vi "仪器初始化.vi"(8 "错误输入（无错误）":errorcluster, 11 "仪器地址":T1) -> (0 "error out":errorcluster, 3 "仪器实例 out":T2)   [LabVIEW 2021]
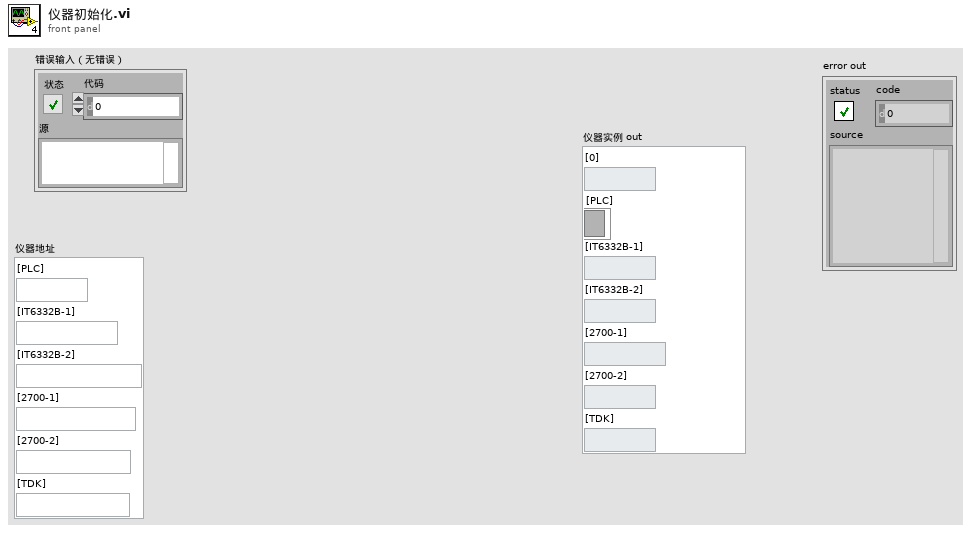
[diagram p1: front panel]
types:
  T1 = typedef "仪器地址输入.ctl" = cluster{"[PLC]":string, "[IT6332B-1]":string, "[IT6332B-2]":string, "[2700-1]":string, "[2700-2]":string, "[TDK]":string}
  T2 = typedef "仪器实例.ctl" = cluster{"[0]":string, "[PLC]":refnum<k24>, "[IT6332B-1]":string, "[IT6332B-2]":string, "[2700-1]":string, "[2700-2]":string, "[TDK]":string}
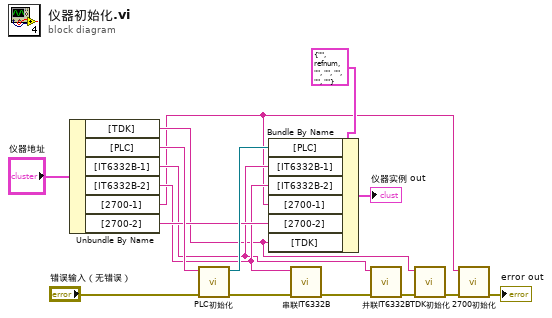
[diagram p0: block diagram]
diagram:
  n1 = Unbundle By Name("仪器地址") -> ("[TDK]"=w5:string, "[PLC]"=w13:string, "[IT6332B-1]"=w7:string, "[IT6332B-2]"=w8:string, "[2700-1]"=w1:string, "[2700-2]"=w10:string)
  n2 = call "PLC初始化.vi"("错误输入（无错误）"="错误输入（无错误）", "ipAddress"=w13) -> ("错误输出"=w9:errorcluster, "引用输出"=w12:refnum<k24>)  [unwired: 7 in, 1 out]
  n3 = Bundle By Name(cluster=T2 {"[0]"="", "[PLC]"=refnum, "[IT6332B-1]"="", "[IT6332B-2]"="", "[2700-1]"="", "[2700-2]"="", "[TDK]"=""} ("仪器实例 out"), "[PLC]"=w12, "[IT6332B-1]"=w7, "[IT6332B-2]"=w8, "[2700-1]"=w1, "[2700-2]"=w10, "[TDK]"=w5) -> (→"仪器实例 out":T2)
  n4 = call "串联IT6332B.vi"("error in (no error)"=w9, "VISA resource name"=w8) -> ("错误输出"=w6:errorcluster)  [unwired: 8 in, 1 out]
  n5 = call "并联IT6332B.vi"("error in (no error)"=w6, "VISA resource name"=w7) -> ("错误输出"=w4:errorcluster)  [unwired: 8 in, 1 out]
  n6 = call "TDK初始化.vi"("error in (no error)"=w4, "TDK地址"=w5) -> ("error out"=w3:errorcluster)  [unwired: 8 in, 1 out]
  n7 = call "2700初始化.vi"("error in (no error)"=w3, "VISA resource name"=w1) -> ("error out"=→"error out":errorcluster)  [unwired: 8 in, 1 out]
